vi "Test LIFA.vi"() -> ()   [LabVIEW 2017]
uses:
  <vilib>/LabVIEW Interface for Arduino/Type Defs/Board Type.ctl
  <vilib>/LabVIEW Interface for Arduino/Type Defs/Connection Type.ctl
  <vilib>/LabVIEW Interface for Arduino/Type Defs/Pin Mode.ctl
  <vilib>/LabVIEW Interface for Arduino/LabVIEW Interface for Arduino.lvlib
panel:
  in  "Slide":u8(slide) scale=0.0..100.0
  in  "Knob":u32(knob) scale=0.0..100.0
  in  "Digital I/O Pin 3":u8
  in  "Digital I/O Pin 2":u8
  in  "stop":bool
  in  "Boolean":bool
  out "error out":errorcluster
  in  "Digital I/O Pin":u8
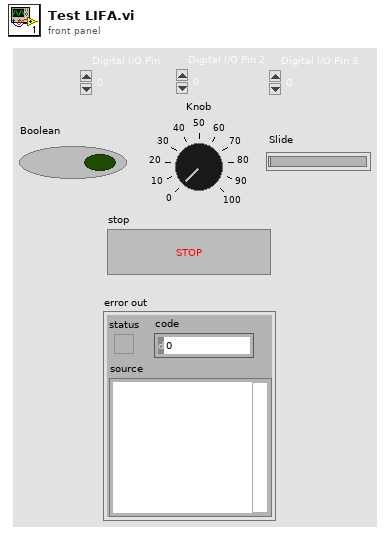
[diagram p1: front panel]
types:
  T1 = typedef "LabVIEW Interface for Arduino.lvlib/Connection Type.ctl" = enum8{"USB / Serial", "XBEE", "BlueSmirf (Bluetooth)"}
  T2 = typedef "LabVIEW Interface for Arduino.lvlib/Board Type.ctl" = enum16{"Uno", "Dimuelanove w/Atmega 328", "Mega 2560"}
  T3 = typedef "LabVIEW Interface for Arduino.lvlib/Arduino Resource.ctl" = cluster{"VISA resource":refnum<visa-resource-name>, "Board Type":T2, "Connection Type":enum8{"USB / Serial"}, "Bytes Per Packet (15)":u8}
  T4 = typedef "LabVIEW Interface for Arduino.lvlib/Pin Mode.ctl" = enum8{"Input", "Output"}
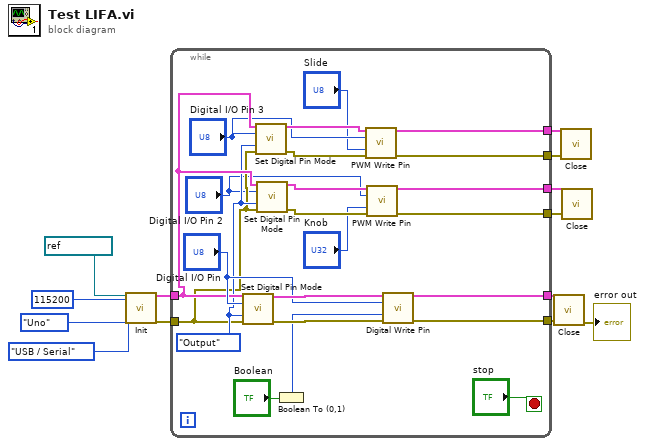
[diagram p0: block diagram]
diagram:
  n1 = call <vilib>:"Init.vi"("VISA resource"=refnum<visa-resource-name> "COM10", "Baud Rate (115200)"=u32 115200, "Board Type (Uno)"=Board_Type."Uno", "Connection Type (USB/Serial)"=Connection_Type."USB / Serial") -> ("Arduino Resource"=w9:T3, "error out"=w8:errorcluster)  [unwired: 14 in]
  n2 = while {
    tunnel: w9 -> [w27]
    tunnel: w8 -> [w25]
    tunnel: [w34] -> w7
    tunnel: [w33] -> w6
    tunnel: [w19] -> w4
    tunnel: [w18] -> w3
    tunnel: [w17] -> w2
    tunnel: [w16] -> w1
    stop <- "stop" stop-if-true
    w26 = Pin_Mode."Output" ("Pin Mode (Input)")
    n3 = call <vilib>:"Set Digital Pin Mode.vi"("Arduino Resource"=w27, "Digital I/O Pin"="Digital I/O Pin", "Pin Mode (Input)"=w26, "error in"=w25) -> ("Arduino Resource"=w36:T3, "error out"=w35:errorcluster)  [unwired: 10 in]
    n4 = call <vilib>:"Set Digital Pin Mode.vi"("Arduino Resource"=w27, "Digital I/O Pin"="Digital I/O Pin 3", "Pin Mode (Input)"=w26, "error in"=w25) -> ("Arduino Resource"=w28:T3, "error out"=w24:errorcluster)  [unwired: 10 in]
    n5 = call <vilib>:"Set Digital Pin Mode.vi"("Arduino Resource"=w27, "Digital I/O Pin"="Digital I/O Pin 2", "Pin Mode (Input)"=w26, "error in"=w25) -> ("Arduino Resource"=w29:T3, "error out"=w23:errorcluster)  [unwired: 10 in]
    n6 = Boolean To (0,1)(Boolean="Boolean") -> (0, 1=w20:i16)
    n7 = call <vilib>:"PWM Write Pin.vi"("Arduino Resource"=w28, "Duty Cycle (0 - 255)"="Digital I/O Pin 3", "PWM Pin (3)"="Slide", "error in"=w24) -> ("Arduino Resource"=w19:T3, "error out"=w18:errorcluster)  [unwired: 10 in]
    n8 = call <vilib>:"PWM Write Pin.vi"("Arduino Resource"=w29, "Duty Cycle (0 - 255)"="Digital I/O Pin 2", "PWM Pin (3)"="Knob", "error in"=w23) -> ("Arduino Resource"=w17:T3, "error out"=w16:errorcluster)  [unwired: 10 in]
    n9 = call <vilib>:"Digital Write Pin.vi"("Arduino Resource"=w36, "Digital I/O Pin (0)"="Digital I/O Pin", "Value (0)"=w20, "error in"=w35) -> ("Arduino Resource"=w34:T3, "error out"=w33:errorcluster)  [unwired: 10 in]
  }
  n10 = call <vilib>:"Close.vi"("Arduino Resource"=w7, "error in"=w6) -> ("error out"=→"error out":errorcluster)  [unwired: 13 in]
  n11 = call <vilib>:"Close.vi"("Arduino Resource"=w4, "error in"=w3) -> ()  [unwired: 13 in, 1 out]
  n12 = call <vilib>:"Close.vi"("Arduino Resource"=w2, "error in"=w1) -> ()  [unwired: 13 in, 1 out]
